vi "Callback_NavigationComplete.vi"(4 "queue out":refnum<queue>, 5 "Event Data":cluster{"sender":refnum<k24>, "e":refnum<k24>}, 6 "Control Ref":refnum<k24>, 7 "Event Common Data":T1) -> ()   [LabVIEW 2020, in "DP_WebView.lvclass"]
uses:
  DP_WebView.lvclass
  C:/Projects/DependencyViewer/DependencyViewer/DP_WebView_class/data/Microsoft.Web.WebView2.Core.dll
  data/Microsoft.Web.WebView2.Core.dll
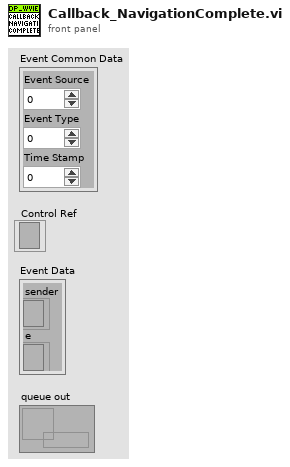
[diagram p1: front panel]
types:
  T1 = cluster{"Event Source":i32, "Event Type":u32, "Time Stamp":u32}
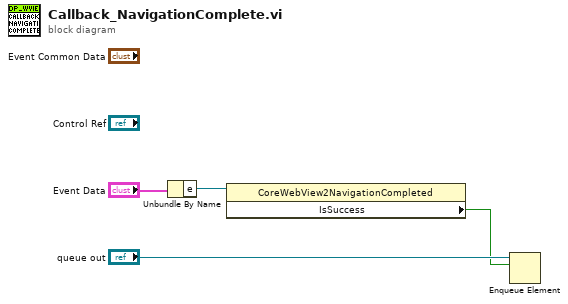
[diagram p0: block diagram]
diagram:
  n1 = Unbundle By Name("Event Data") -> ("e"=w3:refnum<k24>)
  n2 = property class="CoreWebView2NavigationCompleted"(reference=w3) -> ("IsSuccess"=w1:bool)  [unwired: 1 in, 2 out]
  n3 = Enqueue Element(queue="queue out", element=w1) -> ()  [unwired: 2 in, 3 out]
